vi "comp_meas_project.vi"() -> ()   [LabVIEW 2025]
uses:
  <vilib>/Instr/_visa.llb/VISA Configure Serial Port (Instr).vi
panel:
  in  "array type (2D Dbl)":dbl[](array[numeric])
  in  "termination char\n(0xA = '\\n' = LF)":u8=10 format="%.0x"
  in  "stop bits (10: 1 bit)":u16(ring)=10 items=["1.0"=10, "1.5"=15, "2.0"=20]
  in  "data bits (8)":u16=8 min=5 max=8 step=1
  in  "parity (0:none)":enum16{"None", "Odd", "Even", "Mark", "Space"}(ring)
  out "raw reading from serial port":string
  in  "Stop the measurement":bool
  out "Thermometer Sonda [°C}":dbl(graph)
  out "Thermometer Sensor BMP280 [°C]":dbl(graph)
  out "Mode of display:\n0 - BMP280 temp\n1 - BMP280 press\n2 - Sonda temp":dbl
  in  "VISA resource name":refnum<visa-resource-name>
  out "Thermometer Sonda [°C}":dbl(slide) scale=0.0..40.0 scale format="%#_4g"
  out "Air Pressure [hPa]":dbl
  out "Thermometer Sensor BMP280 [°C]":dbl(slide) scale=0.0..40.0 scale format="%#_4g"
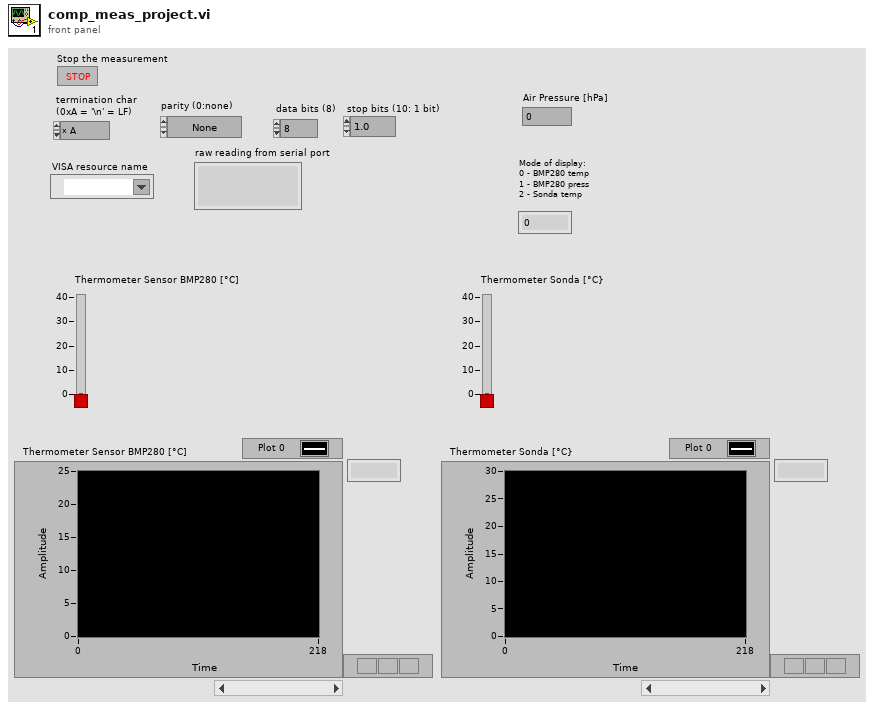
[diagram p1: front panel]
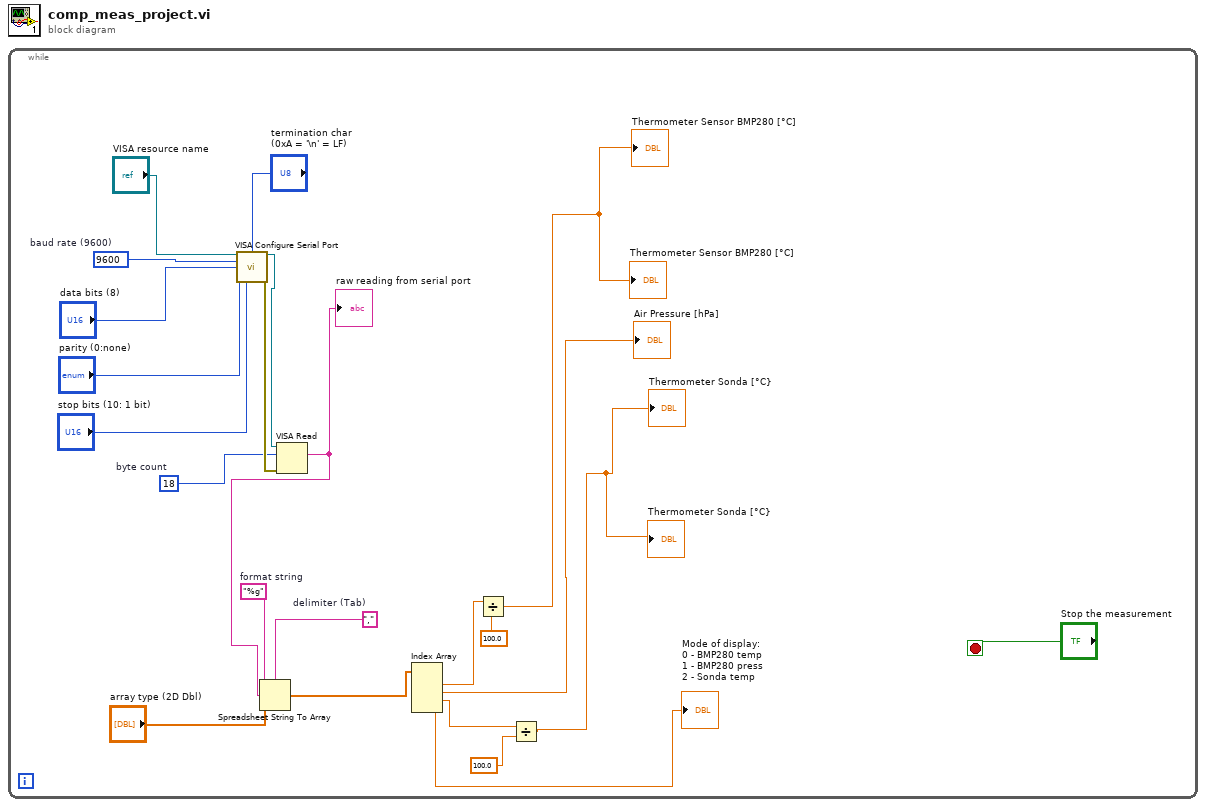
[diagram p0: block diagram]
diagram:
  n1 = while {
    stop <- "Stop the measurement" stop-if-true
    w2 = u32 18  # byte count
    w9 = "%g"  # format string
    w10 = ","  # delimiter (Tab)
    w15 = u32 9600  # baud rate (9600)
    n2 = call-poly "VISA Configure Serial Port"("VISA resource name"="VISA resource name", "termination char\n(0xA = '\\n' = LF)"="termination char\n(0xA = '\\n' = LF)", "baud rate (9600)"=w15, "data bits (8)"="data bits (8)", "parity (0:none)"="parity (0:none)", "stop bits (10: 1 bit)"="stop bits (10: 1 bit)") -> ("VISA resource name out"=w22:refnum<visa-resource-name>, "error out"=w18:errorcluster)  [unwired: 8 in]
    n3 = VISA Read(VISA resource name=w22, byte count=w2, error in (no error)=w18) -> (read buffer=w14:string)  [unwired: 3 out]
    "raw reading from serial port" <- w14
    n4 = Spreadsheet String To Array(delimiter (Tab)=w10, format string=w9, spreadsheet string=w14, array type (2D Dbl)="array type (2D Dbl)") -> (array=w13:dbl[])
    n5 = Index Array "Index Array"(array=w13) -> (element #1=w6:dbl, element #2=→"Air Pressure [hPa]":dbl, element #3=w3:dbl, element #4=→"Mode of display:\n0 - BMP280 temp\n1 - BMP280 press\n2 - Sonda temp":dbl)  [unwired: 4 in]
    n6 = Divide(x=w6, y=100.0) -> (x/y=→"Thermometer Sensor BMP280 [°C]" →"Thermometer Sensor BMP280 [°C]":dbl)
    n7 = Divide(x=w3, y=100.0) -> (x/y=→"Thermometer Sonda [°C}" →"Thermometer Sonda [°C}":dbl)
  }
